vi "MotorStop.vi"(3 "Motor":string="PI1-SHUTTER", 9 "error in (no error)":errorcluster) -> (0 "Motor out":string="PI1-SHUTTER", 6 "error out":errorcluster)   [LabVIEW 2009]
uses:
  Controls/MotorCommand.ctl
  Controls/MotorCommandBasic.ctl
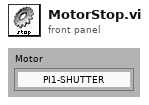
[diagram p1: front panel]
types:
  T1 = typedef "MotorCommandBasic.ctl" = enum16{"SELECT", "MOVE", "PREMOVE", "TURBO", "POS", "NAMED", "INIT", "STOP", "OFF", "SPEED", "QUIT"}
  T2 = typedef "MotorCommand.ctl" = cluster{"Motor":string, "Command":T1, "Movement":i32, "Name":string, "Param":cluster{"VMIN":i32, "VMAX":i32, "ACC":i32}, "Ok?":refnum<k4>, "Go!":refnum<k4>}
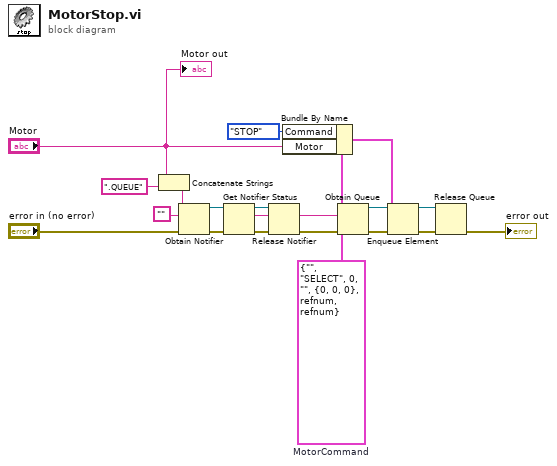
[diagram p0: block diagram]
diagram:
  w17 = T2 {"Motor"="", "Command"=enum."SELECT", "Movement"=0, "Name"="", "Param"={"VMIN"=0, "VMAX"=0, "ACC"=0}, "Ok?"=refnum, "Go!"=refnum}  # MotorCommand
  n1 = Concatenate Strings("Motor", ".QUEUE") -> (w7:string)
  n2 = Obtain Notifier(name (unnamed)=w7, notification data type="", error in (no error)="error in (no error)") -> (notifier out=w8:refnum<notifier>, error out=w9:errorcluster)  [unwired: 1 in, 1 out]
  n3 = Get Notifier Status(notifier=w8, error in (no error)=w9) -> (notifier out=w11:refnum<notifier>, current notification=w3:string, error out=w12:errorcluster)  [unwired: 2 out]
  n4 = Release Notifier(notifier=w11, error in (no error)=w12) -> (error out=w5:errorcluster)  [unwired: 3 out]
  n5 = Bundle By Name(cluster=w17, "Command"=MotorCommandBasic."STOP", "Motor"="Motor") -> (w16:T2)
  n6 = Obtain Queue(name (unnamed)=w3, element data type=w17, error in (no error)=w5) -> (queue out=w19:refnum<queue>, error out=w18:errorcluster)  [unwired: 2 in, 1 out]
  n7 = Enqueue Element(queue=w19, element=w16, error in (no error)=w18) -> (queue out=w13:refnum<queue>, error out=w15:errorcluster)  [unwired: 2 out]
  n8 = Release Queue(queue=w13, error in (no error)=w15) -> (error out=→"error out":errorcluster)  [unwired: 3 out]
  "Motor out" <- "Motor"
